vi "Prax12.2.vi"() -> ()   [LabVIEW 2020]
uses:
  <vilib>/Analysis/NI_AALPro.lvlib
panel:
  out "Algus":dbl
  out "Tõus":dbl
  out "XY Graph":T1(graph)
  out "text":string
  in  "file (use dialog)":path
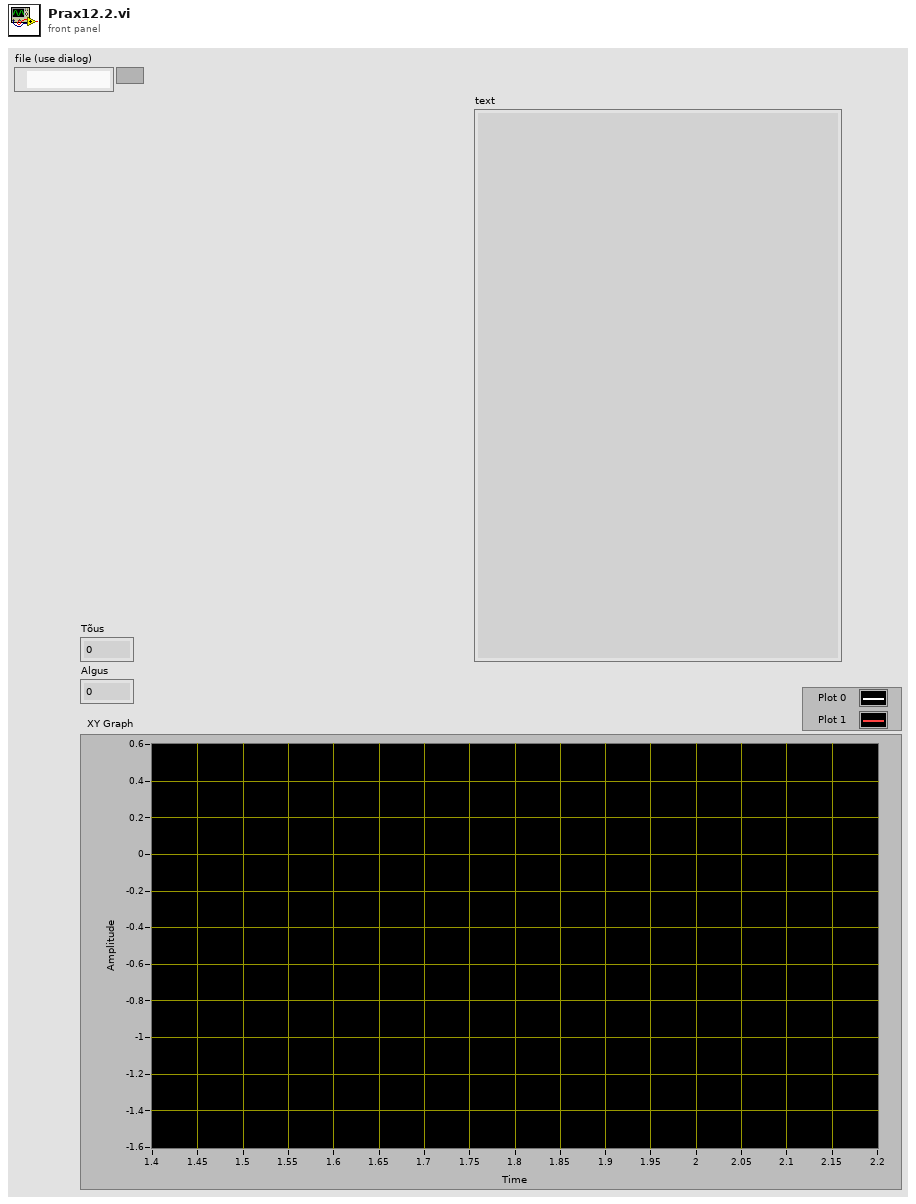
[diagram p1: front panel]
types:
  T1 = cluster{"Best Linear Fit":dbl[], "array type (2D Dbl)":dbl[]}[]
  T2 = cluster{"array type (2D Dbl)":dbl[], "Best Linear Fit":dbl[]}
  T3 = cluster{"array type (2D Dbl)":dbl[], "array type (2D Dbl)":dbl[]}
  T4 = cluster{"array type (2D Dbl)":dbl[], "array type (2D Dbl)":dbl[]}[]
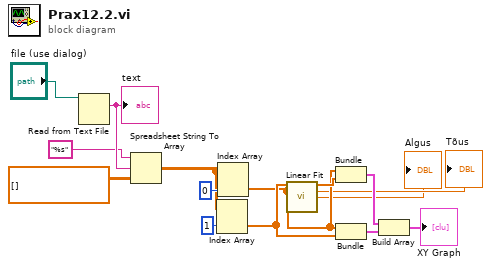
[diagram p0: block diagram]
diagram:
  n1 = Read from Text File(file (use dialog)="file (use dialog)") -> (text=w14:string)  [unwired: 3 in, 3 out]
  "text" <- w14
  n2 = Spreadsheet String To Array(format string="%s", spreadsheet string=w14, array type (2D Dbl)=dbl[][] []) -> (array=w11:dbl[][])  [unwired: 1 in]
  n3 = Index Array(array=w11, index (col)=1 ("disabled index (col)")) -> (element=w7:dbl[])  [unwired: 1 in]
  n4 = Index Array(array=w11, index (col)=0 ("disabled index (col)")) -> (element=w6:dbl[])  [unwired: 1 in]
  n5 = call <vilib>:"Linear Fit.vi"("Y"=w7, "X"=w6) -> ("Best Linear Fit"=w8:dbl[], "slope"=→"Tõus":dbl, "intercept"=→"Algus":dbl)  [unwired: 9 in, 2 out]
  n6 = Bundle("array type (2D Dbl)"=w6, "Best Linear Fit"=w8) -> (w10:T2)  [unwired: 1 in]
  n7 = Bundle("array type (2D Dbl)"=w6, "array type (2D Dbl)"=w7) -> (w9:T3)  [unwired: 1 in]
  n8 = Build Array(w10, w9) -> (→"XY Graph":T4)
